vi "ToTable.vi"(8 "error in":errorcluster, 9 "Table Index (0)":i32, 10 "variant":variant, 11 "Daqmx Module editor node in":refnum<class "DAQmx Module editor node.lvclass">) -> (0 "error out":errorcluster, 1 "row headers":string[](array[string]), 2 "table":string[][](array[string]), 3 "Daqmx Module editor node out":refnum<class "DAQmx Module editor node.lvclass">)   [LabVIEW 2015, in "DAQmx Module editor node.lvclass"]
doc: "Generates the strings needed to display on a table based on the information found in the engine and module configuration classes."
uses:
  DAQmx Module editor node.lvclass
  module/configuration/Daqmx Module configuration.lvclass
  <vilib>/NI/Module Execution Interface/Engine Configuration/engine configuration.lvclass
  module/configuration/Daqmx Module configuration.lvclass/Daqmx Module configuration.ctl
  <vilib>/NI/Configuration Framework/serializable configuration/NISE_CEF_serializable configuration.lvclass/NISE_CEF_serializable configuration.ctl
  <vilib>/NI/Tag Bus/tag/tag descriptor.lvclass/tag descriptor.ctl
  module/configuration/Read Lines.vi
  <vilib>/Utility/LVClass/Get LV Class Name.vi
  <vilib>/NI/Configuration Framework/error generator/NISE_error generator.vi
  <vilib>/NI/Tag Bus Module Framework/channel/TBM channel.lvclass
  <vilib>/NI/Tag Bus/tag/tag descriptor.lvclass
  <vilib>/NI/Configuration Framework/serializable configuration/NISE_CEF_serializable configuration.lvclass
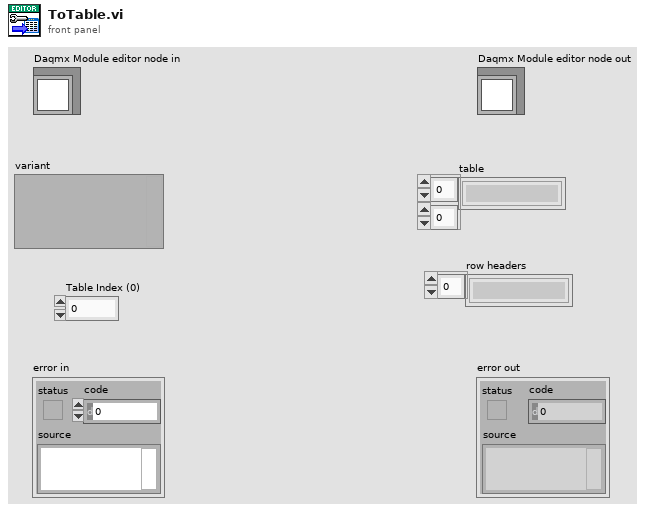
[diagram p1: front panel]
types:
  T1 = typedef "DAQmx Module Configuration.lvclass/Line.ctl" = cluster{"Channel Array":refnum<class "TBM channel.lvclass">[], "Physical Channel":string, "Measurement Type":T2, "Parameters":T3}
  T2 = typedef "DAQmx Module Configuration.lvclass/Measurement Type.ctl" = enum16{"Digital Input", "Digital Output", "Voltage Input", "Voltage Output", "Current Input", "Current Output", "RTD", "Thermocouple", "Strain", "PWM"}
  T3 = typedef "DAQmx Module Configuration.lvclass/Parameters.ctl" = cluster{"Digital Config":cluster{"Invert Lines?":bool}, "Voltage Config":cluster{"Maximum Value (V)":dbl, "Minimum Value (V)":dbl, "in terminal configuration (V)":i32, "out terminal configuration (V)":i32}, "Current Config":cluster{"Maximum Value (A)":dbl, "Minimum Value (A)":dbl, "shunt resistor location":i32, "input terminal configuration (C)":i32, "external shunt resistor value":dbl}, "RTD Config":cluster{"Maximum Value (°C)":dbl, "Minimum Value (°C)":dbl, "resistance configuration":i32, "r0":dbl, "current excitation value":dbl, "rtd type":i32, "current excitation source":i32}, "Thermocouple Config":cluster{"Minimum Value (C)":dbl, "Maximum Value (C)":dbl, "thermocouple type":i32, "cjc source":i32, "cjc value":dbl}, "Strain Config":cluster{"Maximum Value":dbl, "Minimum Value":dbl, "bridge information":cluster{"strain configuration":i32, "lead wire resistance":dbl, "initial bridge voltage":dbl, "voltage excitation source":i32, "voltage excitation value":dbl}, "strain gage information":cluster{"gage factor":dbl, "nominal gage resistance":dbl, "poisson ratio":dbl}}, "PWM Config":cluster{"Idle State":bool}}
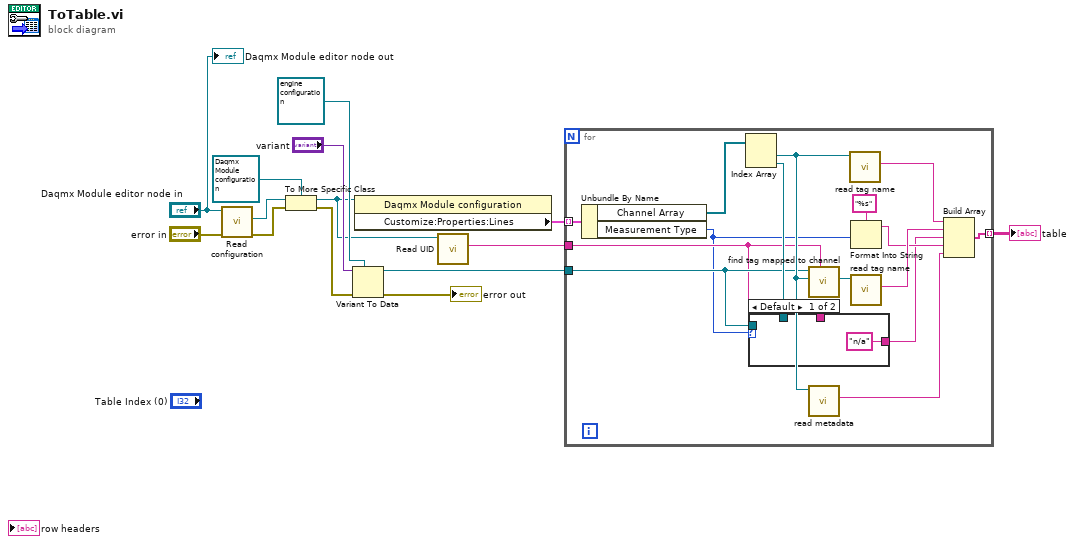
[diagram p0: block diagram]
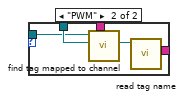
[diagram p2: hidden frame]
diagram:
  n1 = call-dynamic "Read configuration.vi"("error in"="error in", "Daqmx Module editor node in"="Daqmx Module editor node in") -> ("error out"=w14:errorcluster, "configuration"=w1:refnum<class "NISE_CEF_serializable configuration.lvclass">)  [unwired: 7 in, 1 out]
  n2 = To More Specific Class(target class=refnum<class "Daqmx Module configuration.lvclass"> refnum ("tag bus configurable plugin module configuration"), reference=w1, error in=w14) -> (specific class reference=w6:refnum<class "Daqmx Module configuration.lvclass">, error out=w4:errorcluster)
  n3 = Variant To Data(error in=w4, type=refnum<class "engine configuration.lvclass"> refnum ("engine configuration"), Variant="variant") -> (data=w9:refnum<class "engine configuration.lvclass">, error out=→"error out":errorcluster)
  n4 = property class="Daqmx Module configuration"(reference=w6) -> ("Customize:Properties:Lines"=w12:T1[])  [unwired: 1 in, 2 out]
  n5 = call <vilib>:"Read UID.vi"("configuration in"=w6) -> ("instance id"=w5:string)  [unwired: 8 in, 2 out]
  n6 = for {
    tunnel: w12 -> [w29] mode=indexing
    tunnel: w9 -> [w17]
    tunnel: [w26] -> w7 mode=indexing
    tunnel: w5 -> [w16]
    n7 = Unbundle By Name(w29) -> ("Channel Array"=w24:refnum<class "TBM channel.lvclass">[], "Measurement Type"=w15:T2)
    n8 = Index Array(array=w24) -> (element #1=w20:refnum<class "TBM channel.lvclass">, element #2=w18:refnum<class "TBM channel.lvclass">)  [unwired: 2 in]
    n9 = case shown="Default" w15 {
      tunnel: ["n/a" ("name") w34] -> w19
      tunnel: w18 -> [_ w33]
      tunnel: w17 -> [_ w32]
      tunnel: w16 -> [_ w31]
      frame Default {
      }
      frame "PWM" {
        n10 = call <vilib>:"find tag mapped to channel.vi"("owner"=w31, "channel"=w33, "engine configuration in"=w32) -> ("tag"=w35:refnum<class "tag descriptor.lvclass">)  [unwired: 6 in, 2 out]
        n11 = call <vilib>:"read tag name.vi"("system tag in"=w35) -> ("name"=w34:string)  [unwired: 8 in, 2 out]
      }
    }
    n12 = call <vilib>:"find tag mapped to channel.vi"("owner"=w16, "channel"=w20, "engine configuration in"=w17) -> ("tag"=w27:refnum<class "tag descriptor.lvclass">)  [unwired: 6 in, 2 out]
    n13 = call <vilib>:"read metadata.vi"("system tag in"=w20) -> ("metadata"=w23:string)  [unwired: 8 in, 2 out]
    n14 = call <vilib>:"read tag name.vi"("system tag in"=w20) -> ("name"=w28:string)  [unwired: 8 in, 2 out]
    n15 = Format Into String(format string="%s", w15) -> (resulting string=w21:string)  [unwired: 2 in, 1 out]
    n16 = call <vilib>:"read tag name.vi"("system tag in"=w27) -> ("name"=w25:string)  [unwired: 8 in, 2 out]
    n17 = Build Array(w28, w25, w19, w21, w23) -> (w26:string[])
  }
  "table" <- w7
  "Daqmx Module editor node out" <- "Daqmx Module editor node in"
